vi "JogContinuous.vi"(8 "Error In":errorcluster, 10 "direction":i32(ring)=1 items=["Forward"=1, "Backward"=2], 11 "Thorlabs In":refnum<class "Thorlabs.lvclass">) -> (0 "Error Out":errorcluster, 3 "Thorlabs Out":refnum<class "Thorlabs.lvclass">)   [LabVIEW 2018, in "Thorlabs.lvlib" / "Thorlabs.lvclass"]
doc: "This VI moves the tell the Axis to Jog Continiously in the specified direction.\n\nCreator: Slade Jeppesen\nCreated Date: 10/02/20"
uses:
  Thorlabs.lvclass
  Thorlabs.lvclass/Thorlabs.ctl
  C:/AME Test Engineering/LabVIEW/PPLs/Axis/DLLs/ThorLabs.MotionControl.KCube.DCServoCLI.dll
  PPLs/Axis/DLLs/ThorLabs.MotionControl.KCube.DCServoCLI.dll
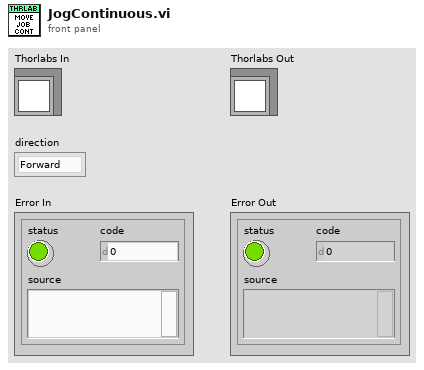
[diagram p1: front panel]
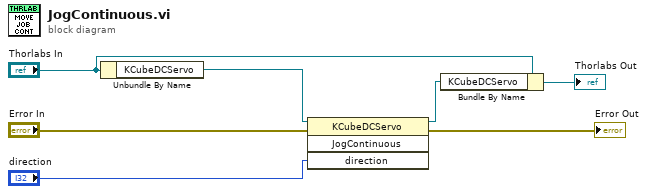
[diagram p0: block diagram]
diagram:
  n1 = Unbundle By Name("Thorlabs In") -> ("KCubeDCServo"=w7:refnum<k24>)
  n2 = invoke class="KCubeDCServo" method="JogContinuous"(reference=w7, error in="Error In", "direction"="direction") -> (reference out=w2:refnum<k24>, error out=→"Error Out":errorcluster)  [unwired: 1 in, 2 out]
  n3 = Bundle By Name(cluster="Thorlabs In", "KCubeDCServo"=w2) -> (→"Thorlabs Out":refnum<class "Thorlabs.lvclass">)
